vi "DrawChessboard.vi"(8 "error in (no error)":errorcluster, 10 "Chessboard Corners Info":T3, 11 "Target Size":T2) -> (0 "error out":errorcluster, 3 "image data":T1)   [LabVIEW 2020, in "feature_detection.lvlib"]
uses:
  feature_detection.lvlib
  Chessboard Corner Info.ctl
  common/Image Size (Integer).ctl
  <vilib>/picture/picture.llb/imagedata.ctl
  common/common.lvlib
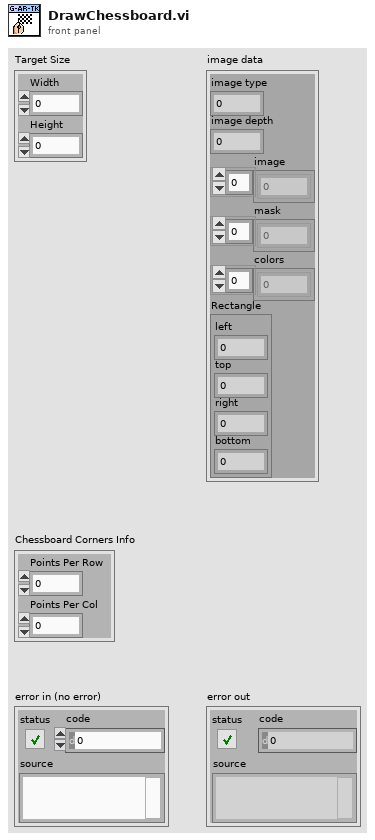
[diagram p1: front panel]
types:
  T1 = typedef "imagedata.ctl" = cluster{"image type":i32, "image depth":i32, "image":u8[], "mask":u8[], "colors":u32[], "Rectangle":cluster{"left":i16, "top":i16, "right":i16, "bottom":i16}}
  T2 = typedef "common.lvlib/Image Size (Integer).ctl" = cluster{"Width":u16, "Height":u16}
  T3 = typedef "feature_detection.lvlib/Chessboard Corner Info.ctl" = cluster{"Points Per Row":u8, "Points Per Col":u8}
  T4 = cluster{"left":i16, "top":i16, "right":i16, "bottom":i16}
  T5 = cluster{"Points Per Row":i32, "Points Per Col":i32}
  T6 = cluster{"left":i32, "top":i32, "right":i32, "bottom":i32}
  T7 = cluster{"Width":i16, "Style":enum32{"Solid", "Dash", "Dot", "DashDot", "DashDotDot"}}
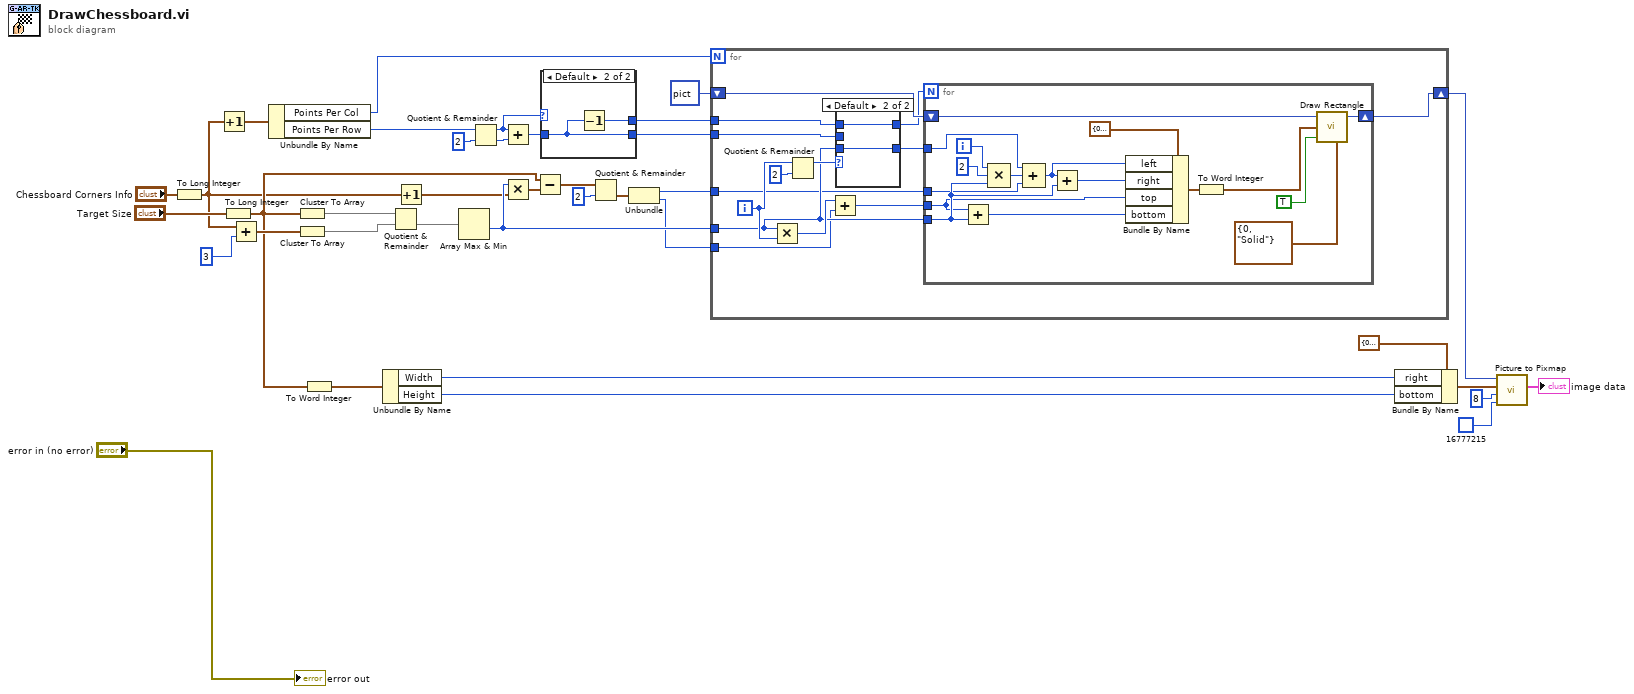
[diagram p0: block diagram]
diagram:
  n1 = To Long Integer(number="Chessboard Corners Info") -> (32bit integer=w1:T5)
  n2 = Increment(x=w1) -> (x+1=w31:T5)
  n3 = To Long Integer(number="Target Size") -> (32bit integer=w6:cluster{"Width":i32, "Height":i32})
  n4 = Add(x=w1, y=u16 3) -> (x+y=w16:T5)
  n5 = Unbundle By Name(w31) -> ("Points Per Col"=w29:i32, "Points Per Row"=w30:i32)
  n6 = Cluster To Array(cluster=w6) -> (array=w7:i32[])
  n7 = Cluster To Array(cluster=w16) -> (array=w8:i32[])
  n8 = To Word Integer(number=w6) -> (16bit integer=w15:cluster{"Width":i16, "Height":i16})
  n9 = Unbundle By Name(w15) -> ("Width"=w23:i16, "Height"=w22:i16)
  n10 = Quotient & Remainder(x=w7, y=w8) -> (floor(x/y)=w35:i32[])  [unwired: 1 out]
  n11 = Increment(x=w1) -> (x+1=w10:T5)
  n12 = Array Max & Min(array=w35) -> (min value=w17:i32)  [unwired: 3 out]
  n13 = Quotient & Remainder(x=w30, y=2) -> (x-y*floor(x/y)=w28:i32, floor(x/y)=w33:i32)
  n14 = Add(x=w28, y=w33) -> (x+y=w5:i32)
  n15 = Multiply(x=w17, y=w10) -> (x*y=w14:T5)
  n16 = Subtract(x=w6, y=w14) -> (x-y=w13:cluster{i32, i32})
  n17 = case shown="Default" w28 {
    tunnel: [w38 w39] -> w27
    tunnel: w5 -> [w38 w39]
    tunnel: [w38 w40] -> w26
    frame 0 {
    }
    frame Default {
      n18 = Decrement(x=w39) -> (x-1=w40:i32)
    }
  }
  n19 = Quotient & Remainder(x=w13, y=2) -> (floor(x/y)=w4:cluster{i32, i32})  [unwired: 1 out]
  n20 = Unbundle(w4) -> (w12:i32, w11:i32)
  n21 = for {
    N: w29 -> [_]
    shift-right: [w48] -> w25
    shift-left: picture data[5B] ("picture") -> [w54]
    tunnel: w27 -> [w46]
    tunnel: w17 -> [w43]
    tunnel: w26 -> [w45]
    tunnel: w12 -> [w42]
    tunnel: w11 -> [w41]
    i -> [w50]
    n22 = Multiply(x=w43, y=w50) -> (x*y=w49:i32)
    n23 = Quotient & Remainder(x=w50, y=2) -> (x-y*floor(x/y)=w52:i32)  [unwired: 1 out]
    n24 = Add(x=w49, y=w41) -> (x+y=w44:i32)
    n25 = case shown="Default" w52 {
      tunnel: w43 -> [_ w57]
      tunnel: [_ w57] -> w51
      tunnel: [w55 w56] -> w47
      tunnel: w46 -> [w55 _]
      tunnel: w45 -> [_ w56]
      frame 0 {
      }
      frame Default {
      }
    }
    n26 = for {
      N: w47 -> [_]
      tunnel: w43 -> [w63]
      shift-right: [w72] -> w48
      shift-left: w54 -> [w74]
      tunnel: w51 -> [w69]
      tunnel: w44 -> [w59]
      tunnel: w42 -> [w58]
      i -> [w68]
      n27 = Add(x=w59, y=w63) -> (x+y=w64:i32)
      n28 = Compound Arithmetic op=MULTIPLY(w68, 2 ("y"), w63) -> (w66:i32)
      n29 = Compound Arithmetic op=ADD(w69, w66, w58) -> (w65:i32)
      n30 = Add(x=w65, y=w63) -> (x+y=w60:i32)
      n31 = Bundle By Name(cluster=T6 {"left"=0, "top"=0, "right"=0, "bottom"=0} ("32bit integer"), "left"=w65, "right"=w60, "top"=w59, "bottom"=w64) -> (w73:T6)
      n32 = To Word Integer(number=w73) -> (16bit integer=w62:T4)
      n33 = call <vilib>:"Draw Rectangle.vi"("picture"=w74, "rect"=w62, "fill?(F)"=TRUE, "pen"=T7 {"Width"=0, "Style"=enum."Solid"}) -> ("new picture"=w72:picture)  [unwired: 5 in]
    }
  }
  n34 = Bundle By Name(cluster=T4 {"left"=0, "top"=0, "right"=0, "bottom"=0} ("rect"), "right"=w23, "bottom"=w22) -> (w9:T4)
  n35 = call <vilib>:"Picture to Pixmap.vi"("Background Color"=u32 16777215, "depth"=8, "rect"=w9, "picture"=w25) -> ("image data"=→"image data":T1)  [unwired: 6 in, 1 out]
  "error out" <- "error in (no error)"
